vi "MIMIC Commands Rev 7.vi"(6 "MIMIC HOST COMMAND":T2(ring)=enum."Read Serial Number", 8 "Input String Data Array":string[](array[string])=["1"], 9 "HWHSflag":bool, 10 "wait (ms)":u32=500, 11 "VISA resource name":refnum<visa-resource-name>="COM5") -> (0 "error out":errorcluster={"status"=FALSE, "code"=1073676294, "source"="VISA Read in MIMIC RecvCommand.vi->MIMIC Commands Rev 2.vi"}, 1 "Receive_buffer":u8[](array[numeric]) format="%x", 2 "Receive_Unpacked_Data":T1)   [LabVIEW 2014]
panel:
  out "local":i32
  out "GUID":string
  out "Array":u8[](array[numeric]) format="%x"
  out "TimeToDecode":u16
  out "VISA resource name OUT":refnum<visa-resource-name>="COM5"
  out "hex integer string":string[](array[string])=["4", "D0", "0", "0", "FF", "2C"]
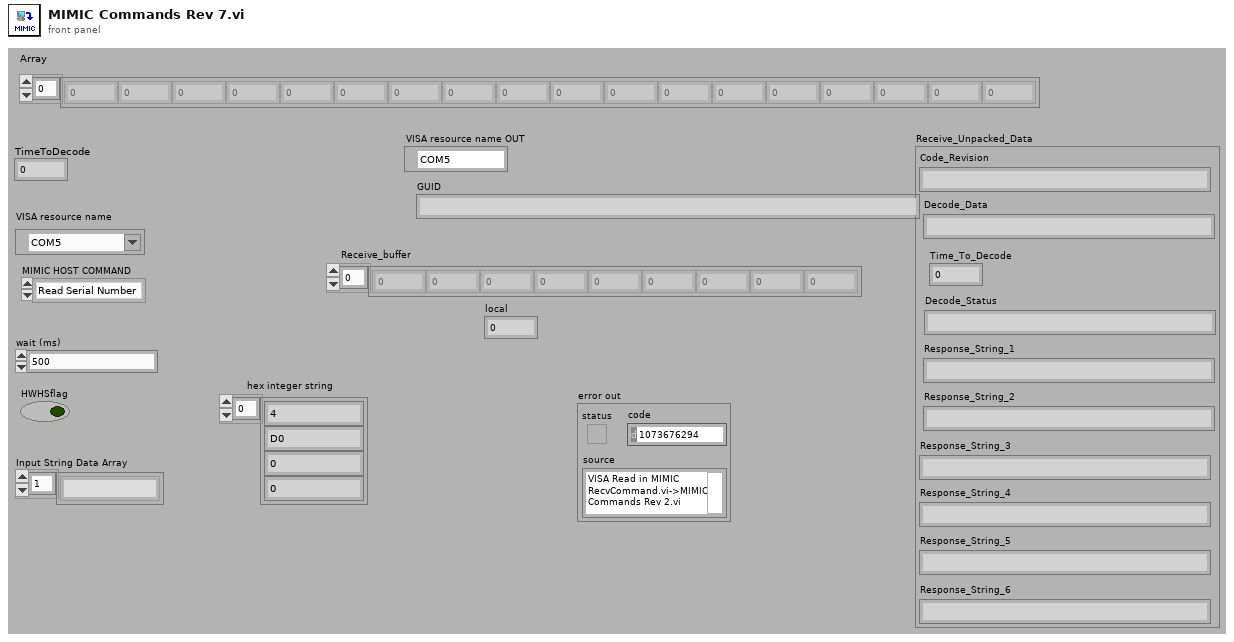
[diagram p1: front panel]
types:
  T1 = cluster{"Code_Revision":string, "Decode_Data":string, "Decode_Status":string, "Response_String_1":string, "Response_String_2":string, "Response_String_3":string, "Response_String_4":string, "Response_String_5":string, "Response_String_6":string, "Time_To_Decode":u16}
  T2 = enum16{"Enter FAT", "Beeper Control", "LED Off", "LED On", "Image Mode", "Start Session", "Stop Session", "Change Buadrate", "Auto Exposure", "Set Manual Exposure", "Read BT Address", "Store BT Address", "Pairing Command", "Query Paired Address", "Pairing Status", "Un-Pairing", "Set Illumination", "Trigger", "Set Defaults", "Imager Time To Decode Test", "Battery Off", "Battery Charge Control", "Read Battery Voltage", "Read Battery Temperature", "Software Version", "StoreFeatureSet", "ReadFeatureSet", "Store Model Number", "Read Model Number", "Store Manufacturing Date", "Read Manufacturing Date", "Store Service Date", "Read Service Date", "Store Serial Number", "Read Serial Number", "Exit FAT", "Read GUID", "Cable Auto ID", "Store RSM 627", "Read RSM 627", "Hall Effect switch", "Store GUID ", "ParamSend", "General", "General-Response", "RSM Init", "RSM EnterFAT", "RSM - SE4500 - Peek PRISM Register GENERIC command", "RSM - SE4500 - Poke PRISM Register GENERIC command", "RSM - SE4500 - GENERIC command", "RSM - SE4500 - GetPDM Calibration", "RSM - SE4500 - SetPDM Calibration", "Get Object Sensor Value", "Store Object Sensor Calibration Value", "Read Object Sensor Calibration Value", "RSM - SE4500 - GetPDM-Z Calibration", "RSM - SE4500 - SetPDM-Z Calibration", "Set-Picklist Calibration", "Get-Picklist Calibration"}
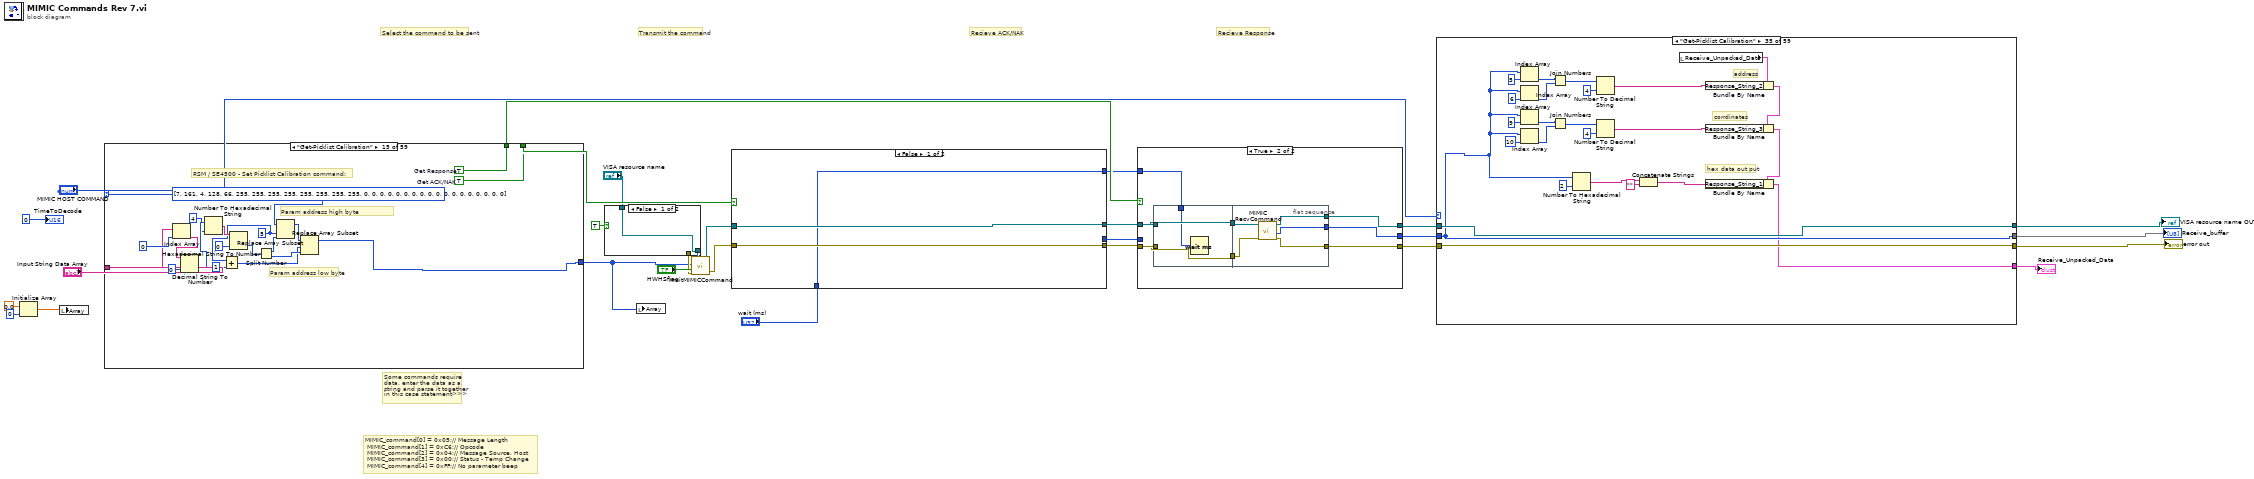
[diagram p0: block diagram]
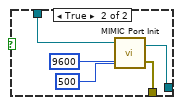
[diagram p2: hidden frame]
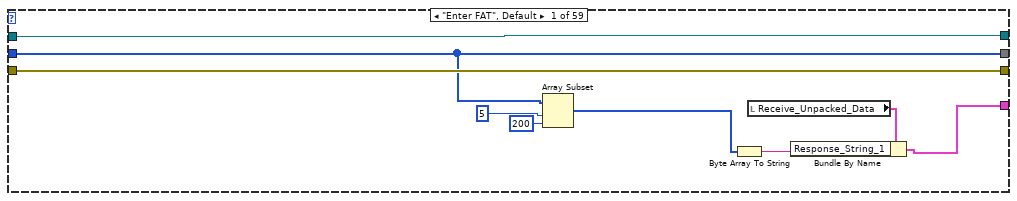
[diagram p3: hidden frame]
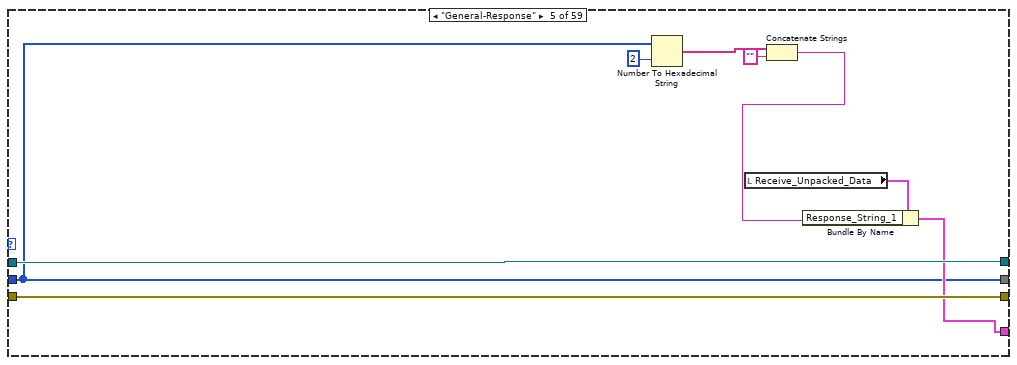
[diagram p7: hidden frame]
diagram:
  # "MIMIC_command[0] = 0x05;// Message Length \n\tMIMIC_command[1] = 0xC6;// Opcode  \n\tMIMIC_command[2] = 0x04;// Message Source, Host \n\tMIMIC_command[3] = 0x00;// Status - Temp Change            \n\tMIMIC_command[4] = 0xFF;// No parameter beep"
  # "Transmit the command"
  # "Recieve Response"
  # "Recieve ACK/NAK"
  # "Select the command to be sent"
  # "Some commands require\ndata, enter the data as a\nstring and parse it together\nin this case statement>>>"
  n1 = Initialize Array(0.0 ("element"), 0 ("dimension size")) -> (w5:dbl[])
  n2 = local write "Array"(w5) -> ()
  n3 = case shown="\"Get-Picklist Calibration\"" "MIMIC HOST COMMAND" {
    tunnel: "Input String Data Array" -> [w37 w39 w62 _ _ _ _ _ w86 w113 w139 w179 w219 w258 w290 w308 _ _ _ w326 w342 w352 w365 w383 w399 _ _ _ _ _ w423 _ _ _ w443 _ _ _ _ w468 _ w480 _ w490 _ _ _ w516 _ w528 _ _ _ _ _ _ _ _ _]
    tunnel: [w31 w45 w66 u8[] [5, 161, 4, 128, 16, 0, 0, 0, 0, 0, 0, 0, 0, 0] u8[] [14, 128, 4, 0, 0, 10, 112, 0, 1, 20, 112, 12, 0, 132] u8[] [14, 128, 4, 0, 0, 10, 112, 0, 1, 20, 112, 31, 0, 113] u8[] [12, 128, 4, 0, 0, 6, 32, 0, 0, 240, 0, 0, 0, 0] u8[] [13, 128, 4, 0, 0, 9, 112, 0, 1, 2, 120, 1, 135, 0] w85 w119 w140 w176 w217 w256 w289 w309 u8[] [4, 228, 4, 0, 0, 0, 0, 0, 0, 0, 0, 0, 0, 0] u8[] [4, 228, 4, 0, 0, 0, 0, 0, 0, 0, 0, 0, 0, 0] u8[] [7, 215, 4, 0, 4, 11, 0, 255, 15, 0, 0, 0, 0, 0] w327 w336 w350 w369 w386 w398 u8[] [16, 161, 4, 128, 16, 0, 0, 0, 0, 0, 0, 0, 0, 0] u8[] [5, 161, 4, 128, 16, 0, 0, 0, 0, 0, 0, 0, 0, 0] u8[] [4, 200, 4, 128, 0, 0, 0, 0, 0, 0, 0, 0, 0, 0] u8[] [5, 161, 4, 128, 25, 0, 0, 0, 0, 0, 0, 0, 0, 0] u8[] [7, 161, 4, 128, 66, 2, 29, 0, 0, 0, 0, 0, 0, 0] w422 u8[] [6, 161, 4, 128, 45, 2, 0, 0, 0, 0, 0, 0, 0, 0] u8[] [7, 161, 4, 128, 48, 19, 136, 0, 0, 0, 0, 0, 0, 0] u8[] [5, 161, 4, 128, 60, 0, 0, 0, 0, 0, 0, 0, 0, 0] w442 u8[] [7, 161, 4, 128, 66, 117, 48, 0, 0, 0, 0, 0, 0, 0] u8[] [7, 161, 4, 128, 66, 117, 49, 0, 0, 0, 0, 0, 0, 0] u8[] [7, 161, 4, 128, 66, 78, 41, 0, 0, 0, 0, 0, 0, 0] u8[] [6, 161, 4, 128, 96, 8] w461 u8[] [7, 161, 4, 128, 66, 3, 36] w482 u8[] [7, 161, 4, 128, 66, 2, 194, 0, 0, 0, 0, 0, 0, 0] w495 u8[] [7, 161, 4, 128, 66, 2, 21, 0, 0, 0, 0, 0, 0, 0] w509 u8[] [7, 161, 4, 128, 66, 2, 23, 0, 0, 0, 0, 0, 0, 0] w521 u8[] [7, 161, 4, 128, 66, 2, 24, 0, 0, 0, 0, 0, 0, 0] w533 u8[] [7, 161, 4, 128, 66, 2, 22, 0, 0, 0, 0, 0, 0, 0] u8[] [5, 161, 4, 128, 54, 254, 160, 0, 0, 0, 0, 0, 0, 0] u8[] [5, 161, 4, 128, 84, 0, 0, 0, 0, 0, 0, 0, 0, 0] u8[] [5, 161, 4, 128, 47] w548 u8[] [5, 161, 4, 128, 110] u8[] [10, 161, 4, 128, 69, 2, 115, 66, 7, 2] u8[] [6, 161, 4, 128, 45, 1, 0, 0, 0, 0, 0, 0, 0, 0] u8[] [7, 161, 4, 128, 66, 2, 115]] -> w6
    tunnel: [w30 w57 w64 w71 w75 w78 w81 w84 w108 w135 w172 w192 w232 w288 w307 w310 w318 w321 w323 w328 w343 w353 w370 w387 w405 w408 w410 w413 w417 w421 w425 w432 w436 w439 w440 w451 w454 w456 w459 w474 w477 w485 w488 w494 w499 w508 w513 w520 w524 w531 w536 w540 w544 w545 w553 w555 w558 w561 w565] -> w25
    tunnel: [w29 w56 w65 w70 w74 w77 w80 w83 w107 w134 w171 w191 w231 w287 w306 w311 w319 w322 w324 w329 w344 w354 w371 w388 w406 w409 w411 w414 w416 w420 w424 w433 w435 w438 w441 w450 w453 w455 w458 w473 w476 w484 w487 w493 w500 w507 w512 w519 w525 w532 w537 w539 w543 w546 w554 w556 w559 w562 w564] -> w27
    frame "LED On" {
      w30 = FALSE  # Get Response
      w29 = TRUE  # Get ACK/NAK
      # "LED data Byte"
      n4 = Index Array(array=w37, index=0) -> (element=w36:string)
      n5 = Decimal String To Number(string=w36) -> (number=w35:i32)  [unwired: 2 in, 1 out]
      n6 = Replace Array Subset(array=u8[] [5, 231, 4, 128, 1, 0, 0, 0, 0, 0, 0, 0, 0, 0], new element=w35, index=4) -> (w31:u8[])
    }
    frame "ParamSend" {
      w57 = FALSE  # Get Response
      w56 = TRUE  # Get ACK/NAK
      n7 = Array Size(array=w39) -> (size(s)=w38:i32)
      n8 = Index Array(array=w39, index=0) -> (element=w61:string)
      n9 = Add(x=w38, y=5) -> (x+y=w43:i32)
      n10 = Hexadecimal String To Number(string=w61) -> (number=w42:u32)  [unwired: 2 in, 1 out]
      n11 = Replace Array Subset(array=u8[] [5, 198, 4, 128, 255, 0, 0, 0, 0, 0, 0, 0, 0, 0], new element=w43, index=0) -> (w54:u8[])
      n12 = Replace Array Subset(array=w54, new element=w42, index=5) -> (w50:u8[])
      n13 = Index Array(array=w39, index=2) -> (element=w49:string)
      n14 = Index Array(array=w39, index=1) -> (element=w53:string)
      n15 = Hexadecimal String To Number(string=w49) -> (number=w40:u32)  [unwired: 2 in, 1 out]
      n16 = Hexadecimal String To Number(string=w53) -> (number=w41:u32)  [unwired: 2 in, 1 out]
      n17 = Replace Array Subset(array=w50, new element=w41, index=6) -> (w46:u8[])
      n18 = Replace Array Subset(array=w46, new element=w40, index=7) -> (w45:u8[])
    }
    frame "Beeper Control" {
      w64 = FALSE  # Get Response
      w65 = TRUE  # Get ACK/NAK
      # "Beeper data Byte"
      n19 = Decimal String To Number(string=w62, offset=0) -> (number=w69:i32[])  [unwired: 1 in, 1 out]
      n20 = Replace Array Subset(array=u8[] [5, 230, 4, 128, 0, 0, 0, 0, 0, 0, 0, 0, 0, 0], new element=w69, index=4) -> (w66:u8[])
    }
    frame "Enter FAT" {
      w71 = TRUE  # Get Response
      w70 = TRUE  # Get ACK/NAK
      # "Enter FAT command:\n0x05:0xA1:0x40:0x80:0x10"
    }
    frame "RSM - SE4500 - GetPDM Calibration" {
      w75 = TRUE  # Get Response
      w74 = FALSE  # Get ACK/NAK
      # "RSM GetDPMCalibration Command"
    }
    frame "RSM - SE4500 - GetPDM-Z Calibration" {
      w78 = TRUE  # Get Response
      w77 = FALSE  # Get ACK/NAK
      # "RSM GetDPMCalibration Command"
    }
    frame "RSM Init" {
      w81 = TRUE  # Get Response
      w80 = FALSE  # Get ACK/NAK
      # "Init RSM command:\n0x0C:0x80:0x04:0x00:0x00:0x06:0x20:0x00:0x00:0xF0"
    }
    frame "RSM EnterFAT" {
      w84 = TRUE  # Get Response
      w83 = FALSE  # Get ACK/NAK
      # "RSM / SE4500 - Enter FAT command:\n0x0D:0x80:0x04:0x00:0x00:0x09:0x70:0x00:0x01:0x02:0x78:0x01:0x87:"
    }
    frame "RSM - SE4500 - Peek PRISM Register GENERIC command" {
      w108 = TRUE  # Get Response
      w107 = FALSE  # Get ACK/NAK
      # "Register Word - HEX String"
      # "RSM / SE4500 - Peek PRISM Register GENERIC command:\n0x0E:0x80:0x04:0x00:0x00:0x0B:0x70:0x00:0x01:0x02:0xC3:0xXX:0xXX:0xXX:0xCS"
      n21 = Index Array(array=w86, index=0) -> (element=w90:string)
      n22 = Hexadecimal String To Number(string=w90, default (0uL)=i16 0 ("default (0 I32)")) -> (number=w88:i16)  [unwired: 1 in, 1 out]
      n23 = Split Number(x=w88) -> (hi(x)=w94:u8, lo(x)=w92:u8)
      n24 = Replace Array Subset(array=u8[] [15, 128, 4, 0, 0, 11, 112, 0, 1, 3, 195, 0, 0, 0, 0], new element=w94, index=11) -> (w91:u8[])
      n25 = Replace Array Subset(array=w91, new element=w92, index=12) -> (w87:u8[])
      n26 = Array Subset(array=w87, index=10, length=3) -> (w97:u8[])
      n27 = for {
        N: 3 -> [_]
        tunnel: w97 -> [w111] mode=indexing
        shift-right: [w109] -> w103
        shift-left: u16 0 -> [w110]
        n28 = Add(x=w110, y=w111) -> (x+y=w109:u16)
      }
      n29 = Not(x=w103) -> (.not. x?=w102:u16)
      n30 = Increment(x=w102) -> (x+1=w101:u16)
      n31 = Replace Array Subset(array=w87, new element=w101, index=13) -> (w85:u8[])
    }
    frame "RSM - SE4500 - GENERIC command" {
      w114 = 1 ("index")
      w118 = 0 ("index")
      w135 = TRUE  # Get Response
      w134 = FALSE  # Get ACK/NAK
      # "Register Word - HEX String"
      # "RSM / SE4500 - Peek PRISM Register GENERIC command:\n0x0E:0x80:0x04:0x00:0x00:0x0B:0x70:0x00:0x01:0x02:0xXX:0xXX:0xXX:0xCS"
      n32 = Index Array(array=w113, index=w118) -> (element=w121:string)
      n33 = Index Array(array=w113, index=w114) -> (element=w115:string)
      n34 = Hexadecimal String To Number(string=w121, default (0uL)=w118) -> (number=w116:i32)  [unwired: 1 in, 1 out]
      n35 = Hexadecimal String To Number(string=w115, default (0uL)=w114) -> (number=w112:i32)  [unwired: 1 in, 1 out]
      n36 = Replace Array Subset(array=u8[] [13, 128, 4, 0, 0, 9, 112, 0, 1, 2, 255, 0, 0], new element=w116, index=10) -> (w122:u8[])
      n37 = Replace Array Subset(array=w122, new element=w112, index=11) -> (w120:u8[])
      n38 = Array Subset(array=w120, index=10, length=2) -> (w125:u8[])
      n39 = for {
        N: 2 -> [_]
        tunnel: w125 -> [w138] mode=indexing
        shift-right: [w136] -> w131
        shift-left: u16 0 -> [w137]
        n40 = Add(x=w137, y=w138) -> (x+y=w136:u16)
      }
      n41 = Not(x=w131) -> (.not. x?=w130:u16)
      n42 = Increment(x=w130) -> (x+1=w129:u16)
      n43 = Replace Array Subset(array=w120, new element=w129, index=12) -> (w119:u8[])
    }
    frame "RSM - SE4500 - Poke PRISM Register GENERIC command" {
      w172 = TRUE  # Get Response
      w171 = FALSE  # Get ACK/NAK
      # "Register Word - HEX String"
      # "Register Word - HEX String"
      # "Value Byte - Decimal String"
      # "RSM / SE4500 - Poke PRISM Register GENERIC command:\n0x0E:0x80:0x04:0x00:0x00:0x0B:0x70:0x00:0x01:0x02:0xC0:0xXX:0xXX:0xXX:0xCS"
      n44 = Index Array(array=w139, index=0) -> (element=w154:string)
      n45 = Index Array(array=w139, index=1) -> (element=w145:string)
      n46 = Hexadecimal String To Number(string=w154, default (0uL)=i16 0 ("default (0 I32)")) -> (number=w152:i16)  [unwired: 1 in, 1 out]
      n47 = Split Number(x=w152) -> (hi(x)=w158:u8, lo(x)=w156:u8)
      n48 = Hexadecimal String To Number(string=w145, default (0uL)=i16 0 ("default (0 I32)")) -> (number=w151:i16)  [unwired: 1 in, 1 out]
      n49 = Replace Array Subset(array=u8[] [16, 128, 4, 0, 0, 12, 112, 0, 1, 2, 151, 0, 0, 0, 0, 0], new element=w158, index=12) -> (w155:u8[])
      n50 = Split Number(x=w151) -> (hi(x)=w148:u8, lo(x)=w150:u8)
      n51 = Replace Array Subset(array=w155, new element=w156, index=11) -> (w143:u8[])
      n52 = Replace Array Subset(array=w143, new element=w148, index=14) -> (w142:u8[])
      n53 = Replace Array Subset(array=w142, new element=w150, index=13) -> (w141:u8[])
      n54 = Array Subset(array=w141, index=10, length=5) -> (w161:u8[])
      n55 = for {
        N: 5 -> [_]
        tunnel: w161 -> [w175] mode=indexing
        shift-right: [w173] -> w167
        shift-left: u16 0 -> [w174]
        n56 = Add(x=w174, y=w175) -> (x+y=w173:u16)
      }
      n57 = Not(x=w167) -> (.not. x?=w166:u16)
      n58 = Increment(x=w166) -> (x+1=w165:u16)
      n59 = Replace Array Subset(array=w141, new element=w165, index=15) -> (w140:u8[])
    }
    frame "RSM - SE4500 - SetPDM Calibration" {
      w192 = TRUE  # Get Response
      w191 = FALSE  # Get ACK/NAK
      # "RSM / SE4500 - SetDPMCalibration command:"
      n60 = for {
        N: 8 -> [_]
        shift-right: [w202] -> w178
        shift-left: u8[] [30, 128, 4, 0, 0, 26, 112, 0, 1, 2, 148, 12, 0, 0, 0, 0, 0, 0, 0, 0, 0, 0, 0, 0, 0, 0, 0, 0, 0, 0, 0] -> [w209]
        tunnel: w179 -> [w208]
        i -> [w204]
        # "high byte"
        # "low byte"
        n61 = Index Array(array=w208, index=w204) -> (element=w197:string)
        n62 = Decimal String To Number(string=w197, default (0L)=0 ("default (0 I32)")) -> (number=w194:i32)  [unwired: 1 in, 1 out]
        n63 = Number To Hexadecimal String(1:i16 4 ("width (-)"), 2:w194) -> (0:w195:string)
        n64 = local read "local"() -> (w200:i32)
        n65 = Hexadecimal String To Number(string=w195, default (0uL)=i16 0 ("default (0 I32)")) -> (number=w210:i16)  [unwired: 1 in, 1 out]
        n66 = Add(x=1 ("y"), y=w200) -> (x+y=w198:i32)
        n67 = Add(x=w204, y=w198) -> (x+y=w201:i32)
        n68 = Add(x=1 ("index"), y=w201) -> (x+y=w206:i32)
        n69 = Split Number(x=w210) -> (hi(x)=w212:u8, lo(x)=w211:u8)
        n70 = Replace Array Subset(array=w209, new element=w212, index=w206) -> (w203:u8[])
        n71 = local write "local"(w198) -> ()
        n72 = Replace Array Subset(array=w203, new element=w211, index=w201) -> (w202:u8[])
      }
      n73 = Array Subset(array=w178, index=10, length=19) -> (w182:u8[])
      n74 = for {
        N: 19 -> [_]
        tunnel: w182 -> [w215] mode=indexing
        shift-right: [w213] -> w188
        shift-left: u16 0 -> [w214]
        n75 = Add(x=w214, y=w215) -> (x+y=w213:u16)
      }
      n76 = Not(x=w188) -> (.not. x?=w187:u16)
      n77 = Increment(x=w187) -> (x+1=w186:u16)
      n78 = Replace Array Subset(array=w178, new element=w186, index=29) -> (w176:u8[])
      "local" <- 12 ("x+y")
    }
    frame "RSM - SE4500 - SetPDM-Z Calibration" {
      w232 = TRUE  # Get Response
      w231 = FALSE  # Get ACK/NAK
      # "RSM / SE4500 - SetDPMCalibration command:"
      n79 = local write "local"(12 ("x+y")) -> ()
      n80 = for {
        N: 8 -> [_]
        shift-right: [w242] -> w218
        shift-left: u8[] [30, 128, 4, 0, 0, 26, 112, 0, 1, 2, 148, 31, 0, 0, 0, 0, 0, 0, 0, 0, 0, 0, 0, 0, 0, 0, 0, 0, 0, 0, 0] -> [w249]
        tunnel: w219 -> [w248]
        i -> [w244]
        # "high byte"
        # "low byte"
        n81 = Index Array(array=w248, index=w244) -> (element=w237:string)
        n82 = Decimal String To Number(string=w237, default (0L)=0 ("default (0 I32)")) -> (number=w234:i32)  [unwired: 1 in, 1 out]
        n83 = Number To Hexadecimal String(1:i16 4 ("width (-)"), 2:w234) -> (0:w235:string)
        n84 = local read "local"() -> (w240:i32)
        n85 = Hexadecimal String To Number(string=w235, default (0uL)=i16 0 ("default (0 I32)")) -> (number=w250:i16)  [unwired: 1 in, 1 out]
        n86 = Add(x=1 ("y"), y=w240) -> (x+y=w238:i32)
        n87 = Add(x=w244, y=w238) -> (x+y=w241:i32)
        n88 = Add(x=1 ("index"), y=w241) -> (x+y=w246:i32)
        n89 = Split Number(x=w250) -> (hi(x)=w252:u8, lo(x)=w251:u8)
        n90 = Replace Array Subset(array=w249, new element=w252, index=w246) -> (w243:u8[])
        n91 = local write "local"(w238) -> ()
        n92 = Replace Array Subset(array=w243, new element=w251, index=w241) -> (w242:u8[])
      }
      n93 = Array Subset(array=w218, index=10, length=19) -> (w222:u8[])
      n94 = for {
        N: 19 -> [_]
        tunnel: w222 -> [w255] mode=indexing
        shift-right: [w253] -> w228
        shift-left: u16 0 -> [w254]
        n95 = Add(x=w254, y=w255) -> (x+y=w253:u16)
      }
      n96 = Not(x=w228) -> (.not. x?=w227:u16)
      n97 = Increment(x=w227) -> (x+1=w226:u16)
      n98 = Replace Array Subset(array=w218, new element=w226, index=29) -> (w217:u8[])
    }
    frame "Set-Picklist Calibration" {
      (unwired) i16 4 ("width (-)")
      w261 = 9 ("index")
      w274 = 5 ("index")
      w288 = TRUE  # Get Response
      w287 = FALSE  # Get ACK/NAK
      # "Param Value high byte"
      # "Param Value low byte"
      # "Param address high byte"
      # "Param address low byte"
      # "RSM / SE4500 - Set Picklist Calibration command:"
      n99 = Index Array(array=w258, index=0 ("default (0 I32)")) -> (element=w281:string)
      n100 = Decimal String To Number(string=w281, default (0L)=0 ("default (0 I32)")) -> (number=w278:i32)  [unwired: 1 in, 1 out]
      n101 = Number To Hexadecimal String(1:i16 4 ("width (-)"), 2:w278) -> (0:w279:string)
      n102 = Add(x=w274, y=1 ("index")) -> (x+y=w273:i32)
      n103 = Hexadecimal String To Number(string=w279, default (0uL)=i16 0 ("default (0 I32)")) -> (number=w284:i16)  [unwired: 1 in, 1 out]
      n104 = Split Number(x=w284) -> (hi(x)=w286:u8, lo(x)=w285:u8)
      n105 = Replace Array Subset(array=u8[] [11, 161, 4, 128, 69, 255, 255, 87, 7, 255, 255, 255, 255, 0, 0, 0, 0, 0, 0, 0, 0, 0, 0, 0, 0, 0, 0, 0, 0, 0, 0], new element=w286, index=w274) -> (w282:u8[])
      n106 = Replace Array Subset(array=w282, new element=w285, index=w273) -> (w257:u8[])
      n107 = Index Array(array=w258, index=1 ("default (0 I32)")) -> (element=w266:string)
      n108 = Decimal String To Number(string=w266, default (0L)=0 ("default (0 I32)")) -> (number=w263:i32)  [unwired: 1 in, 1 out]
      n109 = Number To Hexadecimal String(2:w263) -> (0:w264:string)  [unwired: 1 in]
      n110 = Add(x=w261, y=1 ("index")) -> (x+y=w260:i32)
      n111 = Hexadecimal String To Number(string=w264, default (0uL)=i16 0 ("default (0 I32)")) -> (number=w269:i16)  [unwired: 1 in, 1 out]
      n112 = Split Number(x=w269) -> (hi(x)=w271:u8, lo(x)=w270:u8)
      n113 = Replace Array Subset(array=w257, new element=w271, index=w261) -> (w267:u8[])
      n114 = Replace Array Subset(array=w267, new element=w270, index=w260) -> (w256:u8[])
    }
    frame "Get-Picklist Calibration" {
      w293 = 5 ("index")
      w307 = TRUE  # Get Response
      w306 = TRUE  # Get ACK/NAK
      # "Param address high byte"
      # "Param address low byte"
      # "RSM / SE4500 - Set Picklist Calibration command:"
      n115 = Index Array(array=w290, index=0 ("default (0 I32)")) -> (element=w300:string)
      n116 = Decimal String To Number(string=w300, default (0L)=0 ("default (0 I32)")) -> (number=w297:i32)  [unwired: 1 in, 1 out]
      n117 = Number To Hexadecimal String(1:i16 4 ("width (-)"), 2:w297) -> (0:w298:string)
      n118 = Add(x=w293, y=1 ("index")) -> (x+y=w292:i32)
      n119 = Hexadecimal String To Number(string=w298, default (0uL)=i16 0 ("default (0 I32)")) -> (number=w303:i16)  [unwired: 1 in, 1 out]
      n120 = Split Number(x=w303) -> (hi(x)=w305:u8, lo(x)=w304:u8)
      n121 = Replace Array Subset(array=u8[] [7, 161, 4, 128, 66, 255, 255, 255, 255, 255, 255, 255, 255, 0, 0, 0, 0, 0, 0, 0, 0, 0, 0, 0, 0, 0, 0, 0, 0, 0, 0], new element=w305, index=w293) -> (w301:u8[])
      n122 = Replace Array Subset(array=w301, new element=w304, index=w292) -> (w289:u8[])
    }
    frame "Image Mode" {
      w310 = FALSE  # Get Response
      w311 = TRUE  # Get ACK/NAK
      # "Image Mode Byte:\n00: Decode\n01: SnapShot\n02: Video\n03: Last Decode\n04: las No Decode"
      n123 = Index Array(array=w308, index=0) -> (element=w316:string)
      n124 = Decimal String To Number(string=w316) -> (number=w315:i32)  [unwired: 2 in, 1 out]
      n125 = Replace Array Subset(array=u8[] [5, 247, 4, 128, 0, 0, 0, 0, 0, 0, 0, 0, 0, 0], new element=w315, index=4) -> (w309:u8[])
    }
    frame "Start Session" {
      w318 = FALSE  # Get Response
      w319 = TRUE  # Get ACK/NAK
      # "Start Session"
    }
    frame "Stop Session" {
      w321 = FALSE  # Get Response
      w322 = TRUE  # Get ACK/NAK
      # "Start Session"
    }
    frame "Change Buadrate" {
      w323 = FALSE  # Get Response
      w324 = FALSE  # Get ACK/NAK
      # "Enter FAT command:\n06: 9600\n08: 38400\n0A: 57600\n0B:115200\n0C:230400"
    }
    frame "Auto Exposure" {
      w328 = FALSE  # Get Response
      w329 = TRUE  # Get ACK/NAK
      # "Auto Exposure:\n00:Disabled\n01: Enabled"
      n126 = Index Array(array=w326, index=0) -> (element=w334:string)
      n127 = Decimal String To Number(string=w334) -> (number=w333:i32)  [unwired: 2 in, 1 out]
      n128 = Replace Array Subset(array=u8[] [8, 198, 4, 0, 255, 240, 41, 0, 0, 0, 0, 0, 0, 0], new element=w333, index=7) -> (w327:u8[])
    }
    frame "Set Manual Exposure" {
      w343 = FALSE  # Get Response
      w344 = TRUE  # Get ACK/NAK
      # "Image Mode Byte:\n00: Decode\n01: SnapShot\n02: Video\n03: Last Decode\n04: las No Decode"
      n129 = Index Array(array=w342, index=0) -> (element=w348:string)
      n130 = Decimal String To Number(string=w348, default (0L)=u16 0 ("default (0 I32)")) -> (number=w341:u16)  [unwired: 1 in, 1 out]
      n131 = Split Number(x=w341) -> (hi(x)=w339:u8, lo(x)=w338:u8)
      n132 = Replace Array Subset(array=u8[] [10, 198, 4, 0, 255, 244, 241, 55, 0, 0, 0, 0, 0, 0], new element=w339, index=8) -> (w335:u8[])
      n133 = Replace Array Subset(array=w335, new element=w338, index=9) -> (w336:u8[])
    }
    frame "Store BT Address" {
      w353 = FALSE  # Get Response
      w354 = TRUE  # Get ACK/NAK
      # "Store BT command:\n0x16, 0xA1, 0x04, 0x80, 0x45, 0x02, 0x1D, 0x41, 0x07, 0x42, 0x00, 0x06, 0x00, 0x00, \n\t\t\t\t\t\t\t\t\t\t0x00, 0x00, 0x00, 0x00, 0x00, 0x00,0x00, 0x00, 0xFF, 0xFF};"
      n134 = for {
        N: 6 -> [_]
        tunnel: w352 -> [w363]
        tunnel: [w358] -> w350
        i -> [w360]
        n135 = Index Array(array=w363, index=w360) -> (element=w357:string)
        n136 = Add(x=14 ("index"), y=w360) -> (x+y=w361:i32)
        n137 = Hexadecimal String To Number(string=w357, offset=0) -> (number=w355:u32)  [unwired: 1 in, 1 out]
        n138 = local read "Array"() -> (w359:u8[])
        n139 = Replace Array Subset(array=w359, new element=w355, index=w361) -> (w358:u8[])
        n140 = local write "Array"(w358) -> ()
      }
      "Array" <- u8[] [22, 161, 4, 128, 69, 2, 29, 65, 7, 66, 0, 6, 0, 0, 0, 0, 0, 0, 0, 0, 255, 255, 255, 0, 0, 0]
    }
    frame "General" {
      w367 = 0 ("offset")
      w370 = FALSE  # Get Response
      w371 = TRUE  # Get ACK/NAK
      # "Gneral FAT command:\n0x16, 0xA1, 0x04, 0x80, 0x45, 0x02, 0x1D, 0x41, 0x07, 0x42, 0x00, 0x06, 0x00, 0x00, \n\t\t\t\t\t\t\t\t\t\t0x00, 0x00, 0x00, 0x00, 0x00, 0x00,0x00, 0x00, 0xFF, 0xFF};"
      n141 = Index Array(array=w365, index=w367) -> (element=w366:string)
      n142 = Hexadecimal String To Number(string=w366, offset=w367) -> (number=w364:u32)  [unwired: 1 in, 1 out]
      n143 = for {
        N: w364 -> [_]
        tunnel: w365 -> [w380]
        tunnel: [w375] -> w369
        i -> [w377]
        n144 = Index Array(array=w380, index=w377) -> (element=w374:string)
        n145 = Add(x=0 ("index"), y=w377) -> (x+y=w378:i32)
        n146 = Hexadecimal String To Number(string=w374, offset=0) -> (number=w372:u32)  [unwired: 1 in, 1 out]
        n147 = local read "Array"() -> (w376:u8[])
        n148 = Replace Array Subset(array=w376, new element=w372, index=w378) -> (w375:u8[])
        n149 = local write "Array"(w375) -> ()
      }
      n150 = local write "Array"(u8[] [22, 0, 0, 0, 0, 0, 0, 0, 0, 0, 0, 0, 0, 0, 0, 0, 0, 0, 0, 0, 0, 0, 0, 0, 0, 0]) -> ()
    }
    frame "General-Response" {
      w382 = 0 ("offset")
      w387 = TRUE  # Get Response
      w388 = TRUE  # Get ACK/NAK
      # "Gneral FAT command:\n0x16, 0xA1, 0x04, 0x80, 0x45, 0x02, 0x1D, 0x41, 0x07, 0x42, 0x00, 0x06, 0x00, 0x00, \n\t\t\t\t\t\t\t\t\t\t0x00, 0x00, 0x00, 0x00, 0x00, 0x00,0x00, 0x00, 0xFF, 0xFF};"
      n151 = Index Array(array=w383, index=w382) -> (element=w381:string)
      n152 = Hexadecimal String To Number(string=w381, offset=w382) -> (number=w384:u32)  [unwired: 1 in, 1 out]
      n153 = for {
        N: w384 -> [_]
        tunnel: w383 -> [w397]
        tunnel: [w392] -> w386
        i -> [w394]
        n154 = Index Array(array=w397, index=w394) -> (element=w391:string)
        n155 = Add(x=0 ("index"), y=w394) -> (x+y=w395:i32)
        n156 = Hexadecimal String To Number(string=w391, offset=0) -> (number=w389:u32)  [unwired: 1 in, 1 out]
        n157 = local read "Array"() -> (w393:u8[])
        n158 = Replace Array Subset(array=w393, new element=w389, index=w395) -> (w392:u8[])
        n159 = local write "Array"(w392) -> ()
      }
      n160 = local write "Array"(u8[] [22, 0, 0, 0, 0, 0, 0, 0, 0, 0, 0, 0, 0, 0, 0, 0, 0, 0, 0, 0, 0, 0, 0, 0, 0, 0]) -> ()
    }
    frame "Pairing Command" {
      w405 = TRUE  # Get Response
      w406 = FALSE  # Get ACK/NAK
      # "Pairing  command:\n10 9E 04 80 00 00 02 03 06 08  01 0B 03 00 0F 0F FE 8E"
      n161 = Index Array(array=w399, index=0) -> (element=w403:string)
      n162 = String To Byte Array(string=w403) -> (unsigned byte array=w401:u8[])
      n163 = Replace Array Subset(array=u8[] [16, 158, 4, 128, 0, 0, 0, 0, 0, 8, 1, 11, 3, 0, 15, 15], new element=w401, index=4) -> (w398:u8[])
    }
    frame "Un-Pairing" {
      w408 = TRUE  # Get Response
      w409 = FALSE  # Get ACK/NAK
      # "Enter FAT command:\n0x05:0xA1:0x40:0x80:0x10"
    }
    frame "Set Illumination" {
      w410 = TRUE  # Get Response
      w411 = FALSE  # Get ACK/NAK
      # "Enter FAT command:\n0x05:0xA1:0x40:0x80:0x10"
    }
    frame "Set Defaults" {
      w413 = FALSE  # Get Response
      w414 = TRUE  # Get ACK/NAK
    }
    frame "Exit FAT" {
      w417 = TRUE  # Get Response
      w416 = TRUE  # Get ACK/NAK
    }
    frame "Read BT Address" {
      w421 = TRUE  # Get Response
      w420 = TRUE  # Get ACK/NAK
    }
    frame "LED Off" {
      w425 = FALSE  # Get Response
      w424 = TRUE  # Get ACK/NAK
      # "LED data Byte"
      n164 = Index Array(array=w423, index=0) -> (element=w430:string)
      n165 = Decimal String To Number(string=w430) -> (number=w429:i32)  [unwired: 2 in, 1 out]
      n166 = Replace Array Subset(array=u8[] [5, 232, 4, 128, 1, 0, 0, 0, 0, 0, 0, 0, 0, 0], new element=w429, index=4) -> (w422:u8[])
    }
    frame "Trigger" {
      w432 = TRUE  # Get Response
      w433 = TRUE  # Get ACK/NAK
    }
    frame "Imager Time To Decode Test" {
      w436 = TRUE  # Get Response
      w435 = TRUE  # Get ACK/NAK
      # "Start Session"
    }
    frame "Battery Off" {
      w439 = FALSE  # Get Response
      w438 = TRUE  # Get ACK/NAK
      # "Enter FAT command:\n0x05:0xA1:0x40:0x80:0x10"
    }
    frame "Battery Charge Control" {
      w440 = FALSE  # Get Response
      w441 = TRUE  # Get ACK/NAK
      # "Battery Charge\n0x06, 0xA1, 0x04, 0x80, 0x3D\n0x00: Disable charging of battery\n0x01: Enable charging of battery\n0x02: Enable Slow charge (Hammer)"
      n167 = Index Array(array=w443, index=0) -> (element=w448:string)
      n168 = Decimal String To Number(string=w448) -> (number=w447:i32)  [unwired: 2 in, 1 out]
      n169 = Replace Array Subset(array=u8[] [6, 161, 4, 128, 61, 0, 0, 0, 0, 0, 0, 0, 0, 0], new element=w447, index=5) -> (w442:u8[])
    }
    frame "Read Battery Voltage" {
      w451 = TRUE  # Get Response
      w450 = FALSE  # Get ACK/NAK
      # "Read Battery Voltage command:\n0x07:0xA1:0x04:0x80:0x42:0x75:0x30"
    }
    frame "Read Battery Temperature" {
      w454 = TRUE  # Get Response
      w453 = FALSE  # Get ACK/NAK
      # "Read Battery Temperature command:\n0x07:0xA1:0x04:0x80:0x42:0x75:0x31"
    }
    frame "Software Version" {
      w456 = TRUE  # Get Response
      w455 = TRUE  # Get ACK/NAK
      # "Software Version command:\n\"0x07, 0xA1, 0x04, 0x80, 0x42, 0x4E, 0x29,\""
    }
    frame "Get Object Sensor Value" {
      w459 = TRUE  # Get Response
      w458 = TRUE  # Get ACK/NAK
      # "Get Object Sensor command:\n\"0x06,0xA1,0x04,0x80,0x60,0x08,\""
    }
    frame "Store Object Sensor Calibration Value" {
      w474 = FALSE  # Get Response
      w473 = TRUE  # Get ACK/NAK
      # "Store Object Sensor Calibration command:\n\"0x0B,0xA1,0x04,0x80,0x45,0x03,0x24,0x57,0x07,CAL H,CAL L"
      n170 = Index Array(array=w468, index=1) -> (element=w463:string)
      n171 = Index Array(array=w468, index=0) -> (element=w471:string)
      n172 = Hexadecimal String To Number(string=w471) -> (number=w464:u32)  [unwired: 2 in, 1 out]
      n173 = Hexadecimal String To Number(string=w463) -> (number=w462:u32)  [unwired: 2 in, 1 out]
      n174 = Replace Array Subset(array=u8[] [11, 161, 4, 128, 69, 3, 36, 87, 7, 0, 0], new element=w464, index=9) -> (w466:u8[])
      n175 = Replace Array Subset(array=w466, new element=w462, index=10) -> (w461:u8[])
    }
    frame "Read Object Sensor Calibration Value" {
      w477 = TRUE  # Get Response
      w476 = TRUE  # Get ACK/NAK
      # "Read Object Sensor Calibration command:\n\"0x07,0xA1,0x04,0x80,0x42,0x03,0x24,\""
    }
    frame "StoreFeatureSet" {
      w485 = FALSE  # Get Response
      w484 = TRUE  # Get ACK/NAK
      # "Store Feature Set command:\n\"0x0A, 0xA1, 0x04, 0x80, 0x45, 0x02, 0xC2, 0x42, 0x07,\n0xFF,//Feature Set Value \n0x00, 0x00}; //checksum\""
      n176 = Hexadecimal String To Number(string=w480, offset=0) -> (number=w478:u32[])  [unwired: 1 in, 1 out]
      n177 = Replace Array Subset(array=u8[] [10, 161, 4, 128, 69, 2, 194, 66, 7, 0, 0, 0, 0, 0], new element=w478, index=9) -> (w482:u8[])
    }
    frame "ReadFeatureSet" {
      w488 = TRUE  # Get Response
      w487 = TRUE  # Get ACK/NAK
      # "0x07, 0xA1, 0x04, 0x80, 0x42, 0x02, 0xC2, 0x00, 0x00};"
      # "Read Feature Set command:\n0x07, 0xA1, 0x04, 0x80, 0x42, 0x02, 0xC2,"
    }
    frame "Store Model Number" {
      w494 = FALSE  # Get Response
      w493 = TRUE  # Get ACK/NAK
      # "StoreModel Number command:\n0x20, 0xA1, 0x04, 0x80, 0x45, 0x02, 0x15, 0x53, 0x07, 0x00, 0x12, 0x00, 0x00,\n\t\t\t\t\t\t\t\t\t\t0x00, 0x00, 0x00, 0x00, 0x00, 0x00, 0x00, 0x00, 0x00,\n\t\t\t\t\t\t\t\t\t\t0x00, 0x00, 0x00, 0x00, 0x00, 0x00, 0x00, 0x00, 0x00,\n\t\t\t\t\t\t\t\t\t\t0x00"
      n178 = Index Array(array=w490, index=0) -> (element=w491:string)
      n179 = String To Byte Array(string=w491) -> (unsigned byte array=w492:u8[])
      n180 = Replace Array Subset(array=u8[] [32, 161, 4, 128, 69, 2, 21, 83, 7, 0, 18, 0, 0, 0, 0, 0, 0, 0, 0, 0, 0, 0, 0, 0, 0, 0, 0, 0, 0, 0, 0, 0, 0], new element=w492, index=13) -> (w495:u8[])
    }
    frame "Read Model Number" {
      w499 = TRUE  # Get Response
      w500 = TRUE  # Get ACK/NAK
      # "ReadModel Number command:\n0x07, 0xA1, 0x04, 0x80, 0x42, 0x02, 0x15,"
    }
    frame "Store Manufacturing Date" {
      w508 = FALSE  # Get Response
      w507 = TRUE  # Get ACK/NAK
      # "Store Manufacturing Date command:\n0x15, 0xA1, 0x04, 0x80, 0x45, 0x02, 0x17, 0x53, 0x07, 0x00, 0x07, 0x00, 0x00,\n\t\t\t\t\t\t\t\t\t\t0x00, 0x00, 0x00, 0x00, 0x00, 0x00, 0x00,\n\t\t\t\t\t\t\t\t\t\t0x00"
      n181 = Get Date/Time In Seconds() -> (seconds since 1Jan1904=w506:timestamp)
      n182 = Format Date/Time String(time format string (%c)="%d%b%y", seconds (now)=w506, UTC format=FALSE) -> (date/time string=w502:string)
      n183 = To Upper Case(1:w502) -> (0:w501:string)
      n184 = String To Byte Array(string=w501) -> (unsigned byte array=w503:u8[])
      n185 = Replace Array Subset(array=u8[] [21, 161, 4, 128, 69, 2, 23, 83, 7, 0, 7, 0, 0, 0, 0, 0, 0, 0, 0, 0, 0, 0], new element=w503, index=13) -> (w509:u8[])
    }
    frame "Read Manufacturing Date" {
      w513 = TRUE  # Get Response
      w512 = TRUE  # Get ACK/NAK
      # "Read Feature Set command:\n0x07, 0xA1, 0x04, 0x80, 0x42, 0x02, 0x17,"
    }
    frame "Store Service Date" {
      w520 = FALSE  # Get Response
      w519 = TRUE  # Get ACK/NAK
      # "StoreService Date command:\n0x15, 0xA1, 0x04, 0x80, 0x45, 0x02, 0x18, 0x53, 0x07, 0x00, 0x07, 0x00, 0x00,\n\t\t\t\t\t\t\t\t\t\t0x00, 0x00, 0x00, 0x00, 0x00, 0x00, 0x00,\n\t\t\t\t\t\t\t\t\t\t0x00"
      n186 = Index Array(array=w516, index=0) -> (element=w518:string)
      n187 = String To Byte Array(string=w518) -> (unsigned byte array=w515:u8[])
      n188 = Replace Array Subset(array=u8[] [21, 161, 4, 128, 69, 2, 24, 83, 7, 0, 7, 0, 0, 0, 0, 0, 0, 0, 0, 0, 0, 0], new element=w515, index=13) -> (w521:u8[])
    }
    frame "Read Service Date" {
      w524 = TRUE  # Get Response
      w525 = TRUE  # Get ACK/NAK
      # "Read Service Date command:\n0x07, 0xA1, 0x04, 0x80, 0x42, 0x02, 0x18,"
    }
    frame "Store Serial Number" {
      w531 = FALSE  # Get Response
      w532 = TRUE  # Get ACK/NAK
      # "Store Serial Number command:\n0x1E, 0xA1, 0x04, 0x80, 0x45, 0x02, 0x16, 0x53, 0x07, 0x00, 0x10, 0x00, 0x00,\n\t\t\t\t\t\t\t\t\t\t0x00, 0x00, 0x00, 0x00, 0x00, 0x00, 0x00, 0x00,\n\t\t\t\t\t\t\t\t\t\t0x00, 0x00, 0x00, 0x00, 0x00, 0x00, 0x00, 0x00,\n\t\t\t\t\t\t\t\t\t\t0x00"
      n189 = Index Array(array=w528, index=0) -> (element=w530:string)
      n190 = String To Byte Array(string=w530) -> (unsigned byte array=w527:u8[])
      n191 = Replace Array Subset(array=u8[] [30, 161, 4, 128, 69, 2, 22, 83, 7, 0, 16, 0, 0, 0, 0, 0, 0, 0, 0, 0, 0, 0, 0, 0, 0, 0, 0, 0, 0, 0, 0, 0, 0], new element=w527, index=13) -> (w533:u8[])
    }
    frame "Read Serial Number" {
      w536 = TRUE  # Get Response
      w537 = TRUE  # Get ACK/NAK
      # "Read Serial Number command:\n0x07, 0xA1, 0x04, 0x80, 0x42, 0x02, 0x16,"
    }
    frame "Pairing Status" {
      w540 = TRUE  # Get Response
      w539 = FALSE  # Get ACK/NAK
      # "Read Serial Number command:\n0x05, 0xA1, 0x04, 0x80, 0x36, 0xFE, 0xA0,"
    }
    frame "Query Paired Address" {
      w544 = TRUE  # Get Response
      w543 = FALSE  # Get ACK/NAK
      # "Read Serial Number command:\n0x05, 0xA1, 0x04, 0x80, 0x54,"
    }
    frame "Read GUID" {
      w545 = TRUE  # Get Response
      w546 = TRUE  # Get ACK/NAK
      # "\"0x05, 0xA1, 0x04, 0x80, 0x2F,\""
    }
    frame "Store GUID " {
      w553 = TRUE  # Get Response
      w554 = FALSE  # Get ACK/NAK
      # "32 bytes 0-9, A-F (0x30 - 0x3F, 0x41 - 0x46)"
      # "Start of Date Bytes"
      # "Store GIUD command:\n0x29:0x80:0x04:0x80:0x00:0x25:0x64:0x00:0x0B:0xXX:0xXX:0xXX:0xXX:0xXX:0xXX:0xXX:0xXX:0xXX:0xXX:0xXX:0xXX:0xXX:0xXX:0xXX:0xXX:0xXX:0xXX:0xXX:0xXX:0xXX:0xXX:0xXX:0xXX:0xXX:0xXX:0xXX:0xXX:0xXX:0xXX:0xXX:0xXX:"
      n192 = call "Generate GUID.vi"() -> ("GUID"=w552:string)  [unwired: 10 in, 1 out]
      "GUID" <- w552
      n193 = String To Byte Array(string=w552) -> (unsigned byte array=w549:u8[])
      n194 = Insert Into Array(array=u8[] [41, 128, 4, 128, 0, 37, 100, 0, 11], index=9, new element=w549) -> (w548:u8[])
    }
    frame "Cable Auto ID" {
      w555 = TRUE  # Get Response
      w556 = TRUE  # Get ACK/NAK
      # "0x05, 0xA1, 0x04, 0x00, 0x6E"
    }
    frame "Store RSM 627" {
      w558 = FALSE  # Get Response
      w559 = TRUE  # Get ACK/NAK
      # "0x0A, 0xA1, 0x04, 0x80, 0x45, 0x02, 0x73, 0x42, 0x07, 0x02"
    }
    frame "Hall Effect switch" {
      w561 = TRUE  # Get Response
      w562 = TRUE  # Get ACK/NAK
    }
    frame "Read RSM 627" {
      w565 = TRUE  # Get Response
      w564 = TRUE  # Get ACK/NAK
      # "\"0x07, 0xA1, 0x04, 0x80, 0x42,0x02,0x73\""
    }
  }
  n195 = case shown="False" TRUE {
    tunnel: [w567 w571] -> w8
    tunnel: [_ w570] -> w7
    tunnel: "VISA resource name" -> [w567 w568]
    frame False {
    }
    frame True {
      n196 = call "MIMIC Port Init.vi"("MIMIC TIMEOUT"=u32 500, "MIMC BAUD"=u32 9600, "MIMIC_PORT"=w568) -> ("error out"=w570:errorcluster, "MIMIC PORT RESOURCE"=w571:refnum<visa-resource-name>)
    }
  }
  n197 = local write "Array"(w6) -> ()
  n198 = call "XmitMIMICCommand.vi"("error in (no error)"=w7, "HWHSflag"="HWHSflag", "Command array"=w6, "VISA resource name"=w8) -> ("error out"=w22:errorcluster, "VISA resource name Out"=w21:refnum<visa-resource-name>)
  n199 = case shown="False" w27 {
    tunnel: [w575 w579] -> w26
    tunnel: w22 -> [w575 w584]
    tunnel: w21 -> [w574 w582]
    tunnel: [w574 w580] -> w24
    tunnel: [_ w578] -> w16
    tunnel: [w573 w577] -> w15
    tunnel: "wait (ms)" -> [w573 w576]
    frame False {
    }
    frame True {
      # "NEED TO CHECK ACK"
      n200 = flat-sequence {
        tunnel: w584 -> [w587]
        tunnel: [w587] -> w583
        tunnel: w582 -> [w586]
        tunnel: [w586] -> w581
        tunnel: [w585] -> w577
        tunnel: w576 -> [w585]
        tunnel: w583 -> [w592]
        tunnel: w581 -> [w591]
        tunnel: [w590] -> w580
        tunnel: [w589] -> w579
        tunnel: [w588] -> w578
        frame #0 {
          n201 = Wait (ms)(milliseconds to wait=w585) -> ()  [unwired: 1 out]
        }
        frame #1 {
          n202 = call "MIMIC RecvCommand.vi"("error in"=w592, "VISA resource name"=w591) -> ("error out"=w589:errorcluster, "Receive_buffer"=w588:u8[], "VISA resource name OUT"=w590:refnum<visa-resource-name>)  [unwired: 2 in, 1 out]
          n203 = Number To Hexadecimal String(2:w588) -> (0:→"hex integer string":string[])  [unwired: 1 in]
        }
      }
    }
  }
  n204 = case shown="True" w25 {
    tunnel: [w596 w603] -> w17
    tunnel: w26 -> [w596 w598]
    tunnel: w24 -> [w595 w600]
    tunnel: [w594 w604] -> w18
    tunnel: [w595 w602] -> w19
    tunnel: w16 -> [w594 _]
    tunnel: w15 -> [_ w597]
    frame False {
    }
    frame True {
      n205 = flat-sequence {
        tunnel: [w607] -> w601
        tunnel: w600 -> [w607]
        tunnel: [w606] -> w599
        tunnel: w598 -> [w606]
        tunnel: w597 -> [w605]
        tunnel: [w612] -> w604
        tunnel: [w611] -> w603
        tunnel: [w610] -> w602
        tunnel: w601 -> [w608]
        tunnel: w599 -> [w609]
        frame #0 {
          n206 = Wait (ms)(milliseconds to wait=w605) -> ()  [unwired: 1 out]
        }
        frame #1 {
          n207 = call "MIMIC RecvCommand.vi"("error in"=w609, "VISA resource name"=w608) -> ("error out"=w611:errorcluster, "Receive_buffer"=w612:u8[], "VISA resource name OUT"=w610:refnum<visa-resource-name>)  [unwired: 2 in, 1 out]
        }
      }
    }
  }
  n208 = case shown="\"Get-Picklist Calibration\"" "MIMIC HOST COMMAND" {
    tunnel: w19 -> [w620 w624 w627 w630 w639 w642 w645 w648 w651 w654 w657 w660 w663 w666 w669 w672 w675 w678 w681 w684 w696 w699 w702 w705 w708 w711 w720 w723 w730 w749 w772 w775 w781 w817 w842 w878 w892 w906 w909 w911 w928 w933 w936 w940 w950 w961 w969 w972 w981 w983 w994 w1005 w1010 w1028 w1031 w1034 w1037 w1042 w1055]
    tunnel: [w620 w624 w627 w630 w639 w642 w645 w648 w651 w654 w657 w660 w663 w666 w669 w672 w675 w678 w681 w684 w696 w699 w702 w705 w708 w711 w720 w723 w730 w749 w772 w775 w781 w817 w842 w878 w892 w906 w909 w911 w928 w933 w936 w940 w950 w961 w969 w972 w981 w983 w994 w1005 w1010 w1028 w1031 w1034 w1037 w1042 w1055] -> w13
    tunnel: w18 -> [w616 w623 w626 w629 w631 w641 w644 w647 w650 w653 w656 w659 w662 w665 w668 w671 w674 w677 w680 w683 w694 w698 w701 w704 w707 w710 w712 w722 w725 w747 w771 w774 w777 w786 w821 w847 w883 w897 w907 w913 w923 w932 w937 w941 w947 w960 w966 w971 w978 w984 w990 w998 w1007 w1023 w1030 w1033 w1036 w1039 w1054]
    tunnel: [w616 w623 w626 w629 w631 w641 w644 w647 w650 w653 w656 w659 w662 w665 w668 w671 w674 w677 w680 w683 w689 w698 w701 w704 w707 w710 w712 w722 w724 w747 w771 w774 w776 w786 w821 w847 w883 w897 w907 w912 w926 w932 w934 w941 w945 w960 w963 w971 w976 w984 w986 w996 w1009 w1022 w1030 w1033 w1036 w1038 w1054] -> w12
    tunnel: w17 -> [w621 w622 w625 w628 w638 w640 w643 w646 w649 w652 w655 w658 w661 w664 w667 w670 w673 w676 w679 w682 w695 w697 w700 w703 w706 w709 w719 w721 w729 w750 w770 w773 w780 w816 w841 w877 w891 w905 w908 w910 w927 w931 w935 w942 w951 w959 w970 w973 w982 w985 w993 w1006 w1011 w1027 w1029 w1032 w1035 w1041 w1053]
    tunnel: [w621 w622 w625 w628 w638 w640 w643 w646 w649 w652 w655 w658 w661 w664 w667 w670 w673 w676 w679 w682 w695 w697 w700 w703 w706 w709 w719 w721 w729 w750 w770 w773 w780 w816 w841 w877 w891 w905 w908 w910 w927 w931 w935 w942 w951 w959 w970 w973 w982 w985 w993 w1006 w1011 w1027 w1029 w1032 w1035 w1041 w1053] -> w11
    tunnel: [w618 _ _ _ w632 _ _ _ _ _ _ _ _ _ _ _ _ _ _ _ w690 _ _ _ _ _ w716 _ _ w752 _ _ _ w787 w818 w848 w879 w893 _ _ w924 _ _ _ w943 w953 w964 _ w974 _ w988 w997 _ w1020 _ _ _ _ _] -> w9
    frame "Enter FAT", Default {
      n209 = Array Subset(array=w616, index=5, length=200) -> (w615:u8[])
      n210 = Byte Array To String(unsigned byte array=w615) -> (string=w619:string)
      n211 = local read "Receive_Unpacked_Data"() -> (w617:T1)
      n212 = Bundle By Name(cluster=w617, "Response_String_1"=w619) -> (w618:T1)
    }
    frame "Beeper Control" {
    }
    frame "ParamSend" {
    }
    frame "General" {
    }
    frame "General-Response" {
      n213 = Number To Hexadecimal String(1:i16 2 ("width (-)"), 2:w631) -> (0:w635:string[])
      n214 = local read "Receive_Unpacked_Data"() -> (w633:T1)
      n215 = Concatenate Strings(w635, "" ("string")) -> (w636:string)
      n216 = Bundle By Name(cluster=w633, "Response_String_1"=w636) -> (w632:T1)
    }
    frame "RSM Init" {
    }
    frame "RSM EnterFAT" {
    }
    frame "RSM - SE4500 - Peek PRISM Register GENERIC command" {
    }
    frame "RSM - SE4500 - Poke PRISM Register GENERIC command" {
    }
    frame "RSM - SE4500 - GENERIC command" {
    }
    frame "RSM - SE4500 - SetPDM Calibration" {
    }
    frame "Set-Picklist Calibration" {
    }
    frame "RSM - SE4500 - SetPDM-Z Calibration" {
    }
    frame "LED On" {
    }
    frame "Image Mode" {
    }
    frame "Start Session" {
    }
    frame "Stop Session" {
    }
    frame "Change Buadrate" {
    }
    frame "Auto Exposure" {
    }
    frame "Set Manual Exposure" {
    }
    frame "Read BT Address" {
      n217 = Array Subset(array=w694, index=14, length=6) -> (w689:u8[])
      n218 = Number To Hexadecimal String(1:i16 2 ("width (-)"), 2:w689) -> (0:w687:string[])
      n219 = local read "Receive_Unpacked_Data"() -> (w691:T1)
      n220 = Concatenate Strings(w687, "" ("string")) -> (w686:string)
      n221 = Bundle By Name(cluster=w691, "Response_String_1"=w686) -> (w690:T1)
    }
    frame "Store BT Address" {
    }
    frame "Pairing Command" {
    }
    frame "Un-Pairing" {
    }
    frame "Set Illumination" {
    }
    frame "Set Defaults" {
    }
    frame "Exit FAT" {
      n222 = Array Subset(array=w712, index=5, length=13) -> (w713:u8[])
      n223 = Byte Array To String(unsigned byte array=w713) -> (string=w718:string)
      n224 = local read "Receive_Unpacked_Data"() -> (w717:T1)
      n225 = Bundle By Name(cluster=w717, "Response_String_1"=w718) -> (w716:T1)
    }
    frame "LED Off" {
    }
    frame "Trigger" {
      n226 = Empty Array?(array=w725) -> (empty?=w726:bool)
      n227 = case shown="False" w726 {
        tunnel: w725 -> [w732 _]
        tunnel: [w731 w738] -> w724
        frame False {
          n228 = Array Subset(array=w732, index=5, length=1) -> (w731:u8[])
        }
        frame True {
          # "If empty, init array and set its values to zero."
          n229 = To Unsigned Byte Integer(number=u8 0) -> (unsigned 8bit integer=w736:u8)
          n230 = Initialize Array(w736, 1 ("dimension size")) -> (w738:u8[])
        }
      }
      n231 = Array Subset(array=w725, index=5, length=1) -> ()  [unwired: 1 out]
    }
    frame "Imager Time To Decode Test" {
      n232 = Byte Array To String(unsigned byte array=w747) -> (string=w763:string)
      n233 = Replace Substring(2:16 ("length (len. of substring)"), 3:0 ("offset (0)"), 5:w763) -> (1:w758:string)  [unwired: 1 in, 1 out]
      n234 = String Length(string=w758) -> (length=w757:i32)
      n235 = Index Array(array=w747, index=5) -> (element=w760:u8)
      n236 = Subtract(x=w757, y=2) -> (x-y=w755:i32)
      n237 = Index Array(array=w747, index=7 ("length")) -> (element=w742:u8)
      n238 = Index Array(array=w747, index=6) -> (element=w745:u8)
      n239 = case shown="1" w760 {
        frame 0, Default {
          n240 = local read "Receive_Unpacked_Data"() -> (w764:T1)
          n241 = Bundle By Name(cluster=w764, "Decode_Status"="No Decode" ("Decode_Data")) -> (w765:T1)
          n242 = local write "Receive_Unpacked_Data"(w765) -> ()
        }
        frame 1 {
          n243 = local read "Receive_Unpacked_Data"() -> (w768:T1)
          n244 = Bundle By Name(cluster=w768, "Decode_Status"="SUCCESS" ("Decode_Data")) -> (w767:T1)
          n245 = local write "Receive_Unpacked_Data"(w767) -> ()
        }
      }
      n246 = Join Numbers(hi=u8 0, lo=w745) -> ((hi.lo)=w740:u16)
      n247 = Join Numbers(hi=w742, lo=u8 0 ("hi")) -> ((hi.lo)=w741:u16)
      n248 = Add(x=w740, y=w741) -> (x+y=w739:u16)
      n249 = local write "TimeToDecode"(w739) -> ()
      n250 = Replace Substring(2:2 ("length (len. of substring)"), 3:w755, 5:w758) -> (1:w753:string)  [unwired: 1 in, 1 out]
      n251 = local read "Receive_Unpacked_Data"() -> (w751:T1)
      n252 = Bundle By Name(cluster=w751, "Decode_Data"=w753, "Time_To_Decode"=w739) -> (w752:T1)
    }
    frame "Battery Off" {
    }
    frame "Battery Charge Control" {
    }
    frame "Read Battery Voltage" {
      # "Voltage (MSB_LSB *.0006*2)"
      # "RESPONSE\nLength Byte:\t0x0D\nOpcode Byte:\t0x21\nSource Byte:\t0x00\nStatus Byte:\t0x80\nSub-opcode Byte:\t0x42\nData Byte 1:\t0x75: Attribute MSB\nData Byte 2:\t0x30: Attribute LSB\nData Byte 3:\t0x57: Attribute is Word ('W') value\nData Byte 4:\t0x01\nData Byte 5:\t0xXX: Battery Voltage MSB\nData Byte 6:\t0xXX: Battery Voltage LSB\nData Byte 7:\t0xFF: Packet Termination\nData Byte 8:\t0xFF: Packet Termination\nChecksum High Byte:\t0xXX\nChecksum Low Byte:\t0xXX"
      n253 = Array Subset(array=w777, index=0, length=15) -> (w776:u8[])
    }
    frame "RSM - SE4500 - GetPDM Calibration" {
      n254 = Index Array(array=w786, index=14) -> (element=w812:u8)
      n255 = Index Array(array=w786, index=16) -> (element=w805:u8)
      n256 = Index Array(array=w786, index=13) -> (element=w813:u8)
      n257 = Index Array(array=w786, index=15) -> (element=w806:u8)
      n258 = Index Array(array=w786, index=18) -> (element=w798:u8)
      n259 = Index Array(array=w786, index=20) -> (element=w792:u8)
      n260 = Index Array(array=w786, index=17) -> (element=w799:u8)
      n261 = Index Array(array=w786, index=19) -> (element=w793:u8)
      n262 = Join Numbers(hi=w812, lo=w813) -> ((hi.lo)=w785:u16)
      n263 = Join Numbers(hi=w805, lo=w806) -> ((hi.lo)=w782:u16)
      n264 = Join Numbers(hi=w798, lo=w799) -> ((hi.lo)=w783:u16)
      n265 = Join Numbers(hi=w792, lo=w793) -> ((hi.lo)=w784:u16)
      n266 = Number To Decimal String(number=w785, width (-)=i16 4) -> (decimal integer string=w811:string)
      n267 = Number To Decimal String(number=w782, width (-)=i16 4) -> (decimal integer string=w804:string)
      n268 = Number To Decimal String(number=w783, width (-)=i16 4) -> (decimal integer string=w797:string)
      n269 = Number To Decimal String(number=w784, width (-)=i16 4) -> (decimal integer string=w791:string)
      n270 = local read "Receive_Unpacked_Data"() -> (w809:T1)
      n271 = Bundle By Name(cluster=w809, "Response_String_1"=w811) -> (w802:T1)
      n272 = Bundle By Name(cluster=w802, "Response_String_2"=w804) -> (w789:T1)
      n273 = Bundle By Name(cluster=w789, "Response_String_3"=w797) -> (w788:T1)
      n274 = Bundle By Name(cluster=w788, "Response_String_4"=w791) -> (w787:T1)
    }
    frame "Get-Picklist Calibration" {
      # "corrdinates"
      # "address"
      # "hex data out put"
      n275 = Index Array(array=w821, index=5) -> (element=w837:u8)
      n276 = Index Array(array=w821, index=9) -> (element=w830:u8)
      n277 = Index Array(array=w821, index=6) -> (element=w838:u8)
      n278 = Index Array(array=w821, index=10) -> (element=w831:u8)
      n279 = Join Numbers(hi=w837, lo=w838) -> ((hi.lo)=w826:u16)
      n280 = Join Numbers(hi=w830, lo=w831) -> ((hi.lo)=w825:u16)
      n281 = Number To Hexadecimal String(1:i16 2 ("width (-)"), 2:w821) -> (0:w823:string[])
      n282 = Number To Decimal String(number=w826, width (-)=i16 4) -> (decimal integer string=w836:string)
      n283 = Number To Decimal String(number=w825, width (-)=i16 4) -> (decimal integer string=w829:string)
      n284 = Concatenate Strings(w823, "" ("string")) -> (w820:string)
      n285 = local read "Receive_Unpacked_Data"() -> (w834:T1)
      n286 = Bundle By Name(cluster=w834, "Response_String_2"=w836) -> (w827:T1)
      n287 = Bundle By Name(cluster=w827, "Response_String_3"=w829) -> (w819:T1)
      n288 = Bundle By Name(cluster=w819, "Response_String_1"=w820) -> (w818:T1)
    }
    frame "RSM - SE4500 - GetPDM-Z Calibration" {
      n289 = Index Array(array=w847, index=14) -> (element=w873:u8)
      n290 = Index Array(array=w847, index=16) -> (element=w866:u8)
      n291 = Index Array(array=w847, index=13) -> (element=w874:u8)
      n292 = Index Array(array=w847, index=15) -> (element=w867:u8)
      n293 = Index Array(array=w847, index=22) -> (element=w859:u8)
      n294 = Index Array(array=w847, index=24) -> (element=w853:u8)
      n295 = Index Array(array=w847, index=21) -> (element=w860:u8)
      n296 = Index Array(array=w847, index=23) -> (element=w854:u8)
      n297 = Join Numbers(hi=w873, lo=w874) -> ((hi.lo)=w846:u16)
      n298 = Join Numbers(hi=w866, lo=w867) -> ((hi.lo)=w843:u16)
      n299 = Join Numbers(hi=w859, lo=w860) -> ((hi.lo)=w844:u16)
      n300 = Join Numbers(hi=w853, lo=w854) -> ((hi.lo)=w845:u16)
      n301 = Number To Decimal String(number=w846, width (-)=i16 4) -> (decimal integer string=w872:string)
      n302 = Number To Decimal String(number=w843, width (-)=i16 4) -> (decimal integer string=w865:string)
      n303 = Number To Decimal String(number=w844, width (-)=i16 4) -> (decimal integer string=w858:string)
      n304 = Number To Decimal String(number=w845, width (-)=i16 4) -> (decimal integer string=w852:string)
      n305 = local read "Receive_Unpacked_Data"() -> (w870:T1)
      n306 = Bundle By Name(cluster=w870, "Response_String_1"=w872) -> (w863:T1)
      n307 = Bundle By Name(cluster=w863, "Response_String_2"=w865) -> (w850:T1)
      n308 = Bundle By Name(cluster=w850, "Response_String_3"=w858) -> (w849:T1)
      n309 = Bundle By Name(cluster=w849, "Response_String_4"=w852) -> (w848:T1)
    }
    frame "Get Object Sensor Value" {
      n310 = Index Array(array=w883, index=5) -> (element=w882:u8)
      n311 = Index Array(array=w883, index=6) -> (element=w881:u8)
      n312 = Number To Hexadecimal String(1:i16 2 ("width (-)"), 2:w882) -> (0:w890:string)
      n313 = Number To Hexadecimal String(1:i16 2 ("width (-)"), 2:w881) -> (0:w886:string)
      n314 = local read "Receive_Unpacked_Data"() -> (w888:T1)
      n315 = Bundle By Name(cluster=w888, "Response_String_1"=w890) -> (w884:T1)
      n316 = Bundle By Name(cluster=w884, "Response_String_2"=w886) -> (w879:T1)
    }
    frame "Read Object Sensor Calibration Value" {
      n317 = Index Array(array=w897, index=9) -> (element=w896:u8)
      n318 = Index Array(array=w897, index=10) -> (element=w895:u8)
      n319 = Number To Hexadecimal String(1:i16 2 ("width (-)"), 2:w896) -> (0:w904:string)
      n320 = Number To Hexadecimal String(1:i16 2 ("width (-)"), 2:w895) -> (0:w900:string)
      n321 = local read "Receive_Unpacked_Data"() -> (w902:T1)
      n322 = Bundle By Name(cluster=w902, "Response_String_1"=w904) -> (w898:T1)
      n323 = Bundle By Name(cluster=w898, "Response_String_2"=w900) -> (w893:T1)
    }
    frame "Store Object Sensor Calibration Value" {
    }
    frame "Read Battery Temperature" {
      # "RESPONSE\nLength Byte:\t0x0D\nOpcode Byte:\t0x21\nSource Byte:\t0x00\nStatus Byte:\t0x80\nSub-opcode Byte:\t0x42\nData Byte 1:\t0x75: Attribute MSB\nData Byte 2:\t0x31: Attribute LSB\nData Byte 3:\t0x57: Attribute is Word ('W') value\nData Byte 4:\t0x01\nData Byte 5:\t0xXX: Battery Temperature MSB\nData Byte 6:\t0xXX: Battery Temperature LSB\nData Byte 7:\t0xFF: Packet Termination\nData Byte 8:\t0xFF: Packet Termination\nChecksum High Byte:\t0xXX\nChecksum Low Byte:\t0xXX"
      n324 = Array Subset(array=w913, index=0, length=15) -> (w912:u8[])
    }
    frame "Software Version" {
      n325 = Array Subset(array=w923, index=32, length=16) -> (w920:u8[])
      n326 = Array Subset(array=w923, index=13, length=16) -> (w926:u8[])
      n327 = Byte Array To String(unsigned byte array=w926) -> (string=w919:string)
      n328 = Byte Array To String(unsigned byte array=w920) -> (string=w918:string)
      n329 = Concatenate Strings(w919, "  " ("string"), w918) -> (w916:string)
      n330 = local read "Receive_Unpacked_Data"() -> (w925:T1)
      n331 = Bundle By Name(cluster=w925, "Code_Revision"=w916) -> (w924:T1)
    }
    frame "StoreFeatureSet" {
    }
    frame "ReadFeatureSet" {
      # "Feature Set Responce:\n0x0C, 0x21, 0x00, 0x00, 0x42, 0x02, 0xC2,0x42,0x01,\n\t\t\t\t\t\t\t\t\t\t\t  \t\t\t  0xff, //FEATURE-SET\n\t\t\t\t\t\t\t\t\t\t\t\t\t\t  0xff,0xff, // packet termination\n\t\t\t\t\t\t\t\t\t\t\t\t\t\t  0x00, 0x00}; //checksum"
      n332 = Array Subset(array=w937, index=9, length=1) -> (w934:u8[])
    }
    frame "Store Model Number" {
    }
    frame "Read Model Number" {
      n333 = Array Subset(array=w947, index=13, length=18) -> (w945:u8[])
      n334 = Byte Array To String(unsigned byte array=w945) -> (string=w946:string)
      n335 = local read "Receive_Unpacked_Data"() -> (w944:T1)
      n336 = Bundle By Name(cluster=w944, "Response_String_1"=w946) -> (w943:T1)
    }
    frame "Store Manufacturing Date" {
      n337 = Get Date/Time In Seconds() -> (seconds since 1Jan1904=w958:timestamp)
      n338 = Format Date/Time String(time format string (%c)="%d%b%y", seconds (now)=w958, UTC format=FALSE) -> (date/time string=w955:string)
      n339 = To Upper Case(1:w955) -> (0:w952:string)
      n340 = local read "Receive_Unpacked_Data"() -> (w954:T1)
      n341 = Bundle By Name(cluster=w954, "Response_String_1"=w952) -> (w953:T1)
    }
    frame "Read Manufacturing Date" {
      n342 = Array Subset(array=w966, index=13, length=7) -> (w963:u8[])
      n343 = Byte Array To String(unsigned byte array=w963) -> (string=w965:string)
      n344 = local read "Receive_Unpacked_Data"() -> (w962:T1)
      n345 = Bundle By Name(cluster=w962, "Response_String_1"=w965) -> (w964:T1)
    }
    frame "Store Service Date" {
    }
    frame "Read Service Date" {
      n346 = Array Subset(array=w978, index=13, length=7) -> (w976:u8[])
      n347 = Byte Array To String(unsigned byte array=w976) -> (string=w977:string)
      n348 = local read "Receive_Unpacked_Data"() -> (w975:T1)
      n349 = Bundle By Name(cluster=w975, "Response_String_1"=w977) -> (w974:T1)
    }
    frame "Store Serial Number" {
    }
    frame "Read Serial Number" {
      n350 = Array Subset(array=w990, index=13, length=16) -> (w986:u8[])
      n351 = Byte Array To String(unsigned byte array=w986) -> (string=w989:string)
      n352 = local read "Receive_Unpacked_Data"() -> (w987:T1)
      n353 = Bundle By Name(cluster=w987, "Response_String_1"=w989) -> (w988:T1)
    }
    frame "Query Paired Address" {
      # "Cradle BT Address"
      # "Pair Status\n0x00: Unpaired \n0x01: Paired"
      n354 = Array Subset(array=w998, index=6, length=6) -> (w1001:u8[])
      n355 = Array Subset(array=w998, index=5, length=1) -> (w996:u8[])
      n356 = local read "Receive_Unpacked_Data"() -> (w995:T1)
      n357 = Byte Array To String(unsigned byte array=w1001) -> (string=w1002:string)
      n358 = Bundle By Name(cluster=w995, "Response_String_1"=w1002) -> (w997:T1)
    }
    frame "Pairing Status" {
      # "Pairing Status\n0x00: Cradle is not paired\n0x01: Cradle is paired"
      n359 = Empty Array?(array=w1007) -> (empty?=w1008:bool)
      n360 = case shown="False" w1008 {
        tunnel: w1007 -> [w1013 _]
        tunnel: [w1012 w1019] -> w1009
        frame False {
          n361 = Array Subset(array=w1013, index=5, length=1) -> (w1012:u8[])
        }
        frame True {
          # "If empty, init array and set its values to zero."
          n362 = To Unsigned Byte Integer(number=u8 0) -> (unsigned 8bit integer=w1017:u8)
          n363 = Initialize Array(w1017, 1 ("dimension size")) -> (w1019:u8[])
        }
      }
    }
    frame "Read GUID" {
      n364 = Array Subset(array=w1023, index=5, length=32) -> (w1022:u8[])
      n365 = Byte Array To String(unsigned byte array=w1022) -> (string=w1026:string)
      n366 = local read "Receive_Unpacked_Data"() -> (w1021:T1)
      n367 = Bundle By Name(cluster=w1021, "Response_String_1"=w1026) -> (w1020:T1)
    }
    frame "Cable Auto ID" {
    }
    frame "Store RSM 627" {
    }
    frame "Store GUID " {
    }
    frame "Hall Effect switch" {
      n368 = Empty Array?(array=w1039) -> (empty?=w1040:bool)
      n369 = case shown="True" w1040 {
        tunnel: w1039 -> [w1046 _]
        tunnel: [w1045 w1052] -> w1038
        frame False {
          n370 = Array Subset(array=w1046, index=5, length=1) -> (w1045:u8[])
        }
        frame True {
          # "If empty, init array and set its values to zero."
          n371 = To Unsigned Byte Integer(number=u8 0) -> (unsigned 8bit integer=w1050:u8)
          n372 = Initialize Array(w1050, 1 ("dimension size")) -> (w1052:u8[])
        }
      }
      n373 = Array Subset(array=w1039, index=5, length=1) -> ()  [unwired: 1 out]
    }
    frame "Read RSM 627" {
    }
  }
  "error out" <- w11
  "Receive_buffer" <- w12
  "VISA resource name OUT" <- w13
  "Receive_Unpacked_Data" <- w9
  "TimeToDecode" <- u16 0 ("TimeToDecode")
